vi "Manuele override.vi"() -> ()   [LabVIEW 2019]
panel:
  in  "kruispunt":string
  out "bericht":string
  in  "STOP":bool
  in  "START":bool
  in  "stop 2":bool
  out "address":u32
  out "port":u16
  in  "stop":bool
  in  "vooruit":bool
  in  "achteruit":bool
  in  "links":bool
  in  "rechts":bool
  in  "linksvooruit":bool
  in  "rechtsvooruit":bool
  in  "rechtsachter":bool
  in  "linksachter":bool
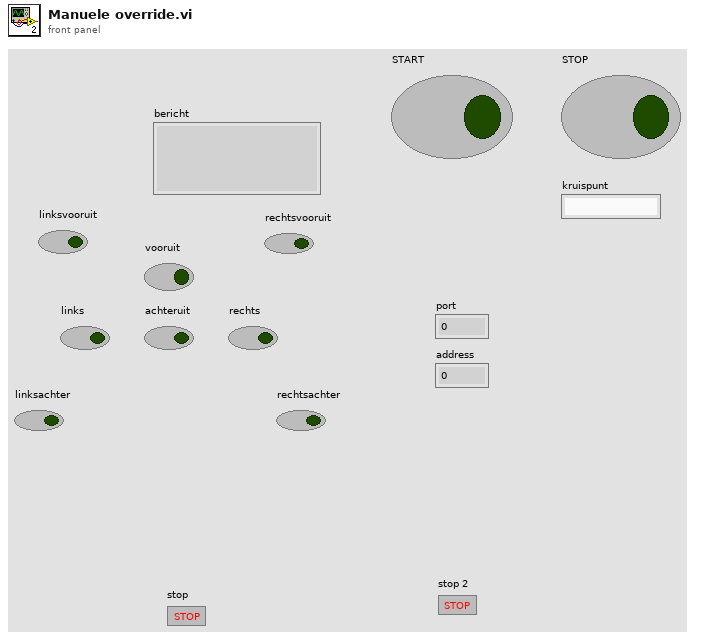
[diagram p1: front panel]
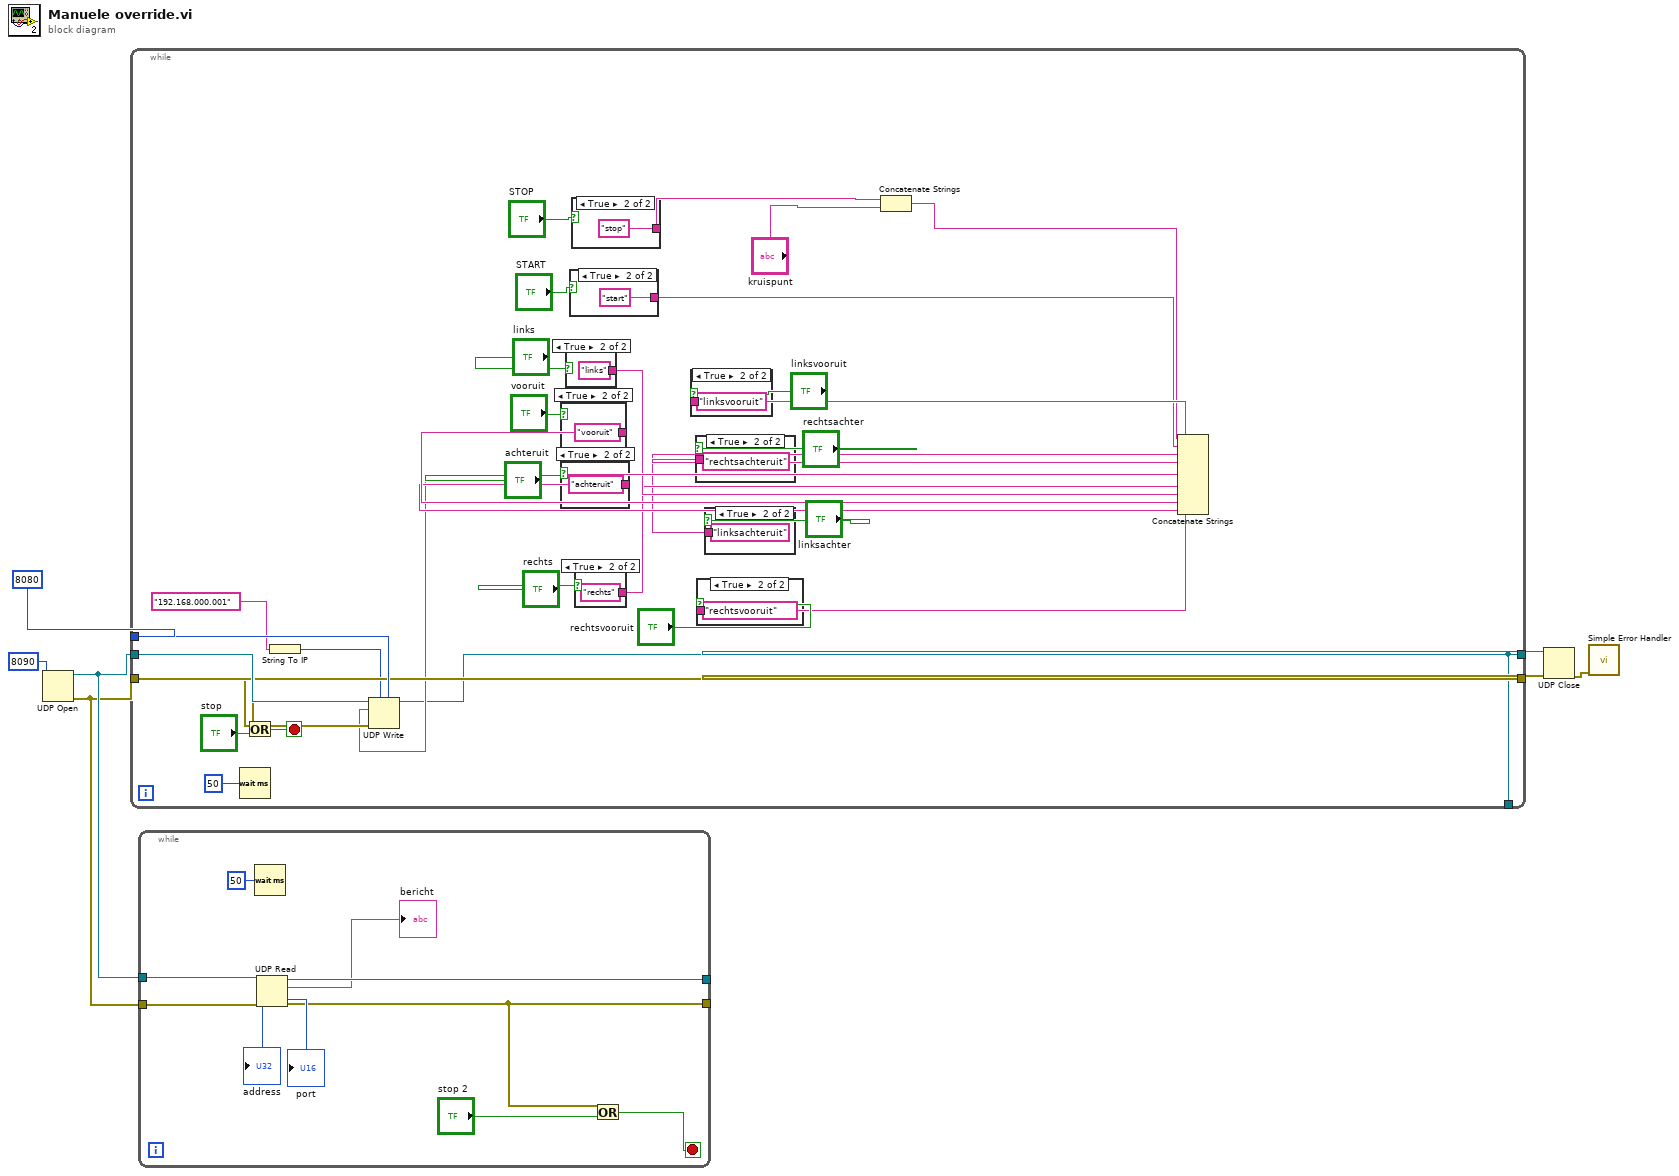
[diagram p0: block diagram]
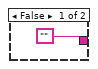
[diagram p2: hidden frame]
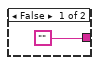
[diagram p3: hidden frame]
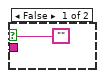
[diagram p4: hidden frame]
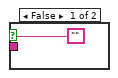
[diagram p5: hidden frame]
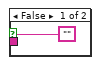
[diagram p6: hidden frame]
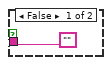
[diagram p7: hidden frame]
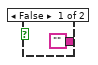
[diagram p8: hidden frame]
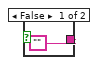
[diagram p9: hidden frame]
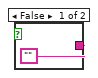
[diagram p10: hidden frame]
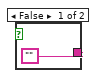
[diagram p11: hidden frame]
diagram:
  n1 = UDP Open(11:8090) -> (port=w3:refnum<k16>, 0:w2:errorcluster)  [unwired: 4 in, 1 out]
  n2 = while {
    tunnel: w3 -> [w40]
    tunnel: w2 -> [w39]
    tunnel: 8080 -> [w35]
    tunnel: [w16] -> w1
    tunnel: [w34] -> w5
    tunnel: [w16] -> _
    stop <- w37 stop-if-true
    n3 = Wait (ms)(milliseconds to wait=50) -> ()  [unwired: 1 out]
    n4 = String To IP(1:"192.168.000.001") -> (0:w27:u32)
    n5 = case shown="True" "vooruit" {
      tunnel: ["" "vooruit"] -> w31
      frame False {
      }
      frame True {
      }
    }
    n6 = case shown="True" "achteruit" {
      tunnel: ["" "achteruit"] -> w30
      frame False {
      }
      frame True {
      }
    }
    n7 = case shown="True" "links" {
      tunnel: ["" "links"] -> w26
      frame False {
      }
      frame True {
      }
    }
    n8 = case shown="True" "START" {
      tunnel: ["" "start"] -> w13
      frame False {
      }
      frame True {
      }
    }
    n9 = case shown="True" "STOP" {
      tunnel: ["" "stop"] -> w9
      frame False {
      }
      frame True {
      }
    }
    n10 = case shown="True" "rechts" {
      tunnel: ["" "rechts"] -> w24
      frame False {
      }
      frame True {
      }
    }
    n11 = case shown="True" "linksvooruit" {
      tunnel: ["" "linksvooruit"] -> w20
      frame False {
      }
      frame True {
      }
    }
    n12 = case shown="True" "rechtsachter" {
      tunnel: ["" "rechtsachteruit"] -> w18
      frame False {
      }
      frame True {
      }
    }
    n13 = case shown="True" "rechtsvooruit" {
      tunnel: ["" "rechtsvooruit"] -> w21
      frame False {
      }
      frame True {
      }
    }
    n14 = case shown="True" "linksachter" {
      tunnel: ["" "linksachteruit"] -> w17
      frame False {
      }
      frame True {
      }
    }
    n15 = Concatenate Strings(w9, "kruispunt") -> (w10:string)
    n16 = Concatenate Strings(w10, w13, w17, w18, w20, w21, w24, w26, w31, w30) -> (w29:string)
    n17 = UDP Write(address=w27, port or service name=w35, connection ID=w40, data in=w29, 8:w39) -> (error out=w34:errorcluster, 3:w16:refnum<k16>)  [unwired: 1 in]
    n18 = Or(x=w34, y="stop") -> (x .or. y?=w37:bool)
  }
  n19 = while {
    tunnel: w3 -> [w70]
    tunnel: w2 -> [w69]
    tunnel: [w66] -> _
    tunnel: [w65] -> _
    stop <- w63 stop-if-true
    n20 = Wait (ms)(milliseconds to wait=u32 50) -> ()  [unwired: 1 out]
    n21 = UDP Read(connection ID=w70, 8:w69) -> (data out=→"bericht":string, error out=w65:errorcluster, 3:w66:refnum<k16>, 4:→"port":u16, 6:→"address":u32)  [unwired: 2 in]
    n22 = Or(x=w65, y="stop 2") -> (x .or. y?=w63:bool)
  }
  n23 = UDP Close(connection ID=w1, 8:w5) -> (error out=w4:errorcluster)  [unwired: 1 out]
  n24 = call <vilib>:"Simple Error Handler.vi"("error in (no error)"=w4) -> ()  [unwired: 4 in, 5 out]
